vi "DownsampleArray.vi"(10 "Number of Samples":i32, 11 "data":sgl[](array[numeric])) -> (3 "values":sgl[](array[numeric]))   [LabVIEW 2017, in "TestPanel.lvlib"]
uses:
  <vilib>/addons/InsightCM/Devices/Shared/Common/TestPanel/TestPanel.lvlib
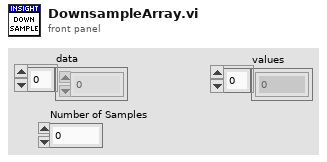
[diagram p1: front panel]
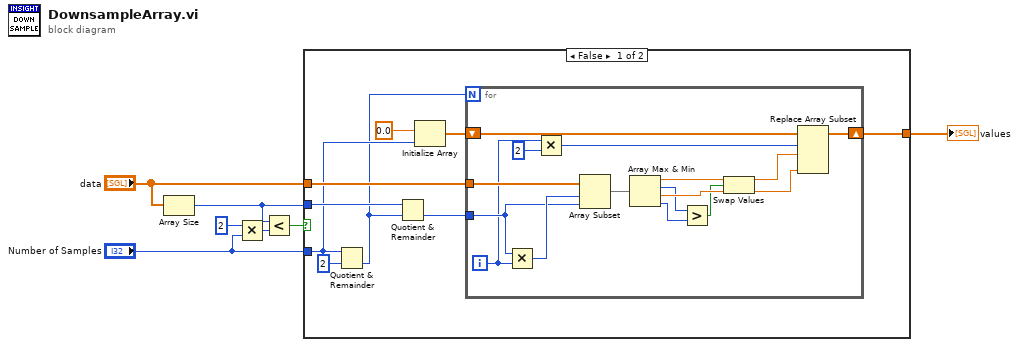
[diagram p0: block diagram]
diagram:
  n1 = Array Size(array="data") -> (size(s)=w1:i32)
  n2 = Multiply(x=2, y="Number of Samples") -> (x*y=w7:i32)
  n3 = Less?(x=w1, y=w7) -> (x < y?=w5:bool)
  n4 = case shown="False" w5 {
    tunnel: [w10 w33] -> w4
    tunnel: "data" -> [w15 w33]
    tunnel: "Number of Samples" -> [w9 _]
    tunnel: w1 -> [w14 _]
    frame False {
      n5 = Quotient & Remainder(x=w9, y=2) -> (floor(x/y)=w8:i32)  [unwired: 1 out]
      n6 = Quotient & Remainder(x=w14, y=w8) -> (floor(x/y)=w13:i32)  [unwired: 1 out]
      n7 = Initialize Array(sgl 0.0, w9) -> (w11:sgl[])
      n8 = for {
        N: w8 -> [_]
        tunnel: w15 -> [w32]
        tunnel: w13 -> [w30]
        shift-right: [w27] -> w10
        shift-left: w11 -> [w28]
        i -> [w18]
        n9 = Multiply(x=w30, y=w18) -> (x*y=w31:i32)
        n10 = Multiply(x=w18, y=2) -> (x*y=w17:i32)
        n11 = Array Subset(array=w32, index=w31, length=w30) -> (w29:sgl[])
        n12 = Array Max & Min(array=w29) -> (max value=w26:sgl, max index (indices)=w24:i32, min value=w25:sgl, min index (indices)=w23:i32)
        n13 = Greater?(x=w24, y=w23) -> (0:w22:bool)
        n14 = Swap Values(12:w26, 13:w22, 14:w25) -> (1:w21:sgl, 3:w20:sgl)
        n15 = Replace Array Subset(array=w28, new element #1=w21, index #1=w17, new element #2=w20) -> (w27:sgl[])  [unwired: 1 in]
      }
    }
    frame True {
    }
  }
  "values" <- w4
